vi "LEDpoi_main.vi"() -> ()   [LabVIEW 2014]
uses:
  typeDefs/location.ctl
  typeDefs/playParams.ctl
  typeDefs/editControl.ctl
  typeDefs/variantFlat.ctl
  typeDefs/editViewPlay.ctl
  typeDefs/loopDataType.ctl
  typeDefs/pictChooser.ctl
  typeDefs/labelInfo.ctl
  typeDefs/jumpTpInfo.ctl
  typeDefs/dimmerInfo.ctl
  typeDefs/cmdQaction.ctl
  typeDefs/pixxelAction.ctl
  <vilib>/Utility/sysdir.llb/System Directory Type.ctl
  typeDefs/parseAction.ctl
  typeDefs/saveDataType.ctl
  typeDefs/pixxelMultiAction.ctl
  <vilib>/picture/picture.llb/Draw True-Color Pixmap.vi
  <userlib>/_OpenG.lib/comparison/comparison.llb/U32 Changed__ogtk.vi
  <vilib>/Utility/file.llb/Read From Spreadsheet File (string).vi
  <userlib>/_OpenG.lib/array/array.llb/Empty 2D Array (String)__ogtk.vi
  <vilib>/Utility/file.llb/Write To Spreadsheet File (string).vi
  <vilib>/Utility/config.llb/NI_LVConfig.lvlib
panel:
  in  "debug":bool
  in  "loopData":T1
  in  "close":bool
  in  "mainTab":enum32{"editor", "Group", "setup", "unused1"}(tab)
  in  "delProg":bool
  in  "reloadProg":bool
  in  "openList":bool
  in  "saveList":bool
  in  "POI-Sequence":i32(listbox)
  in  "deleteProg":bool
  in  "loadProg":bool
  in  "saveProgAs":bool
  in  "activePoi":T5(radio) caption="Poi"
  in  "editArray":T2[](array[typedef])
  in  "editTab":enum32{"play", "LoopStart", "LoopEnd", "Dimmer"}(tab)
  out "Pixel":dbl
  out "2D Picture":picture
  in  "editDefPlay":T6={"delay"=100, "fromFrame"=0, "active"=TRUE, "picIndex"=2, "toFrame"=1, "loops"=0}
  out "Frame":dbl
  in  "labelInfo":T7={"LoopID"=1, "active"=TRUE, "LoopCount"=1} {"LoopCount" min=1 max=254; "LoopID" min=1 max=254}
  in  "loopEndInfo":T8={"LoopID"=1, "active"=TRUE} caption="Jump to..." {"LoopID" min=1 max=254}
  in  "dimmer":T9={"Dimmer Level"=100, "active"=TRUE} caption="Jump to..." {"Dimmer Level" min=1 max=254}
  in  "chooser":T4[](array[typedef])
  in  "uploadAll":bool
  in  "uploadProgOnly":bool
  in  "startProg":bool
  in  "pauseProg":bool
  out "error out":errorcluster
  in  "saveProg":bool
  out "working":bool
  out "status":string
  in  "jumpTo":bool
  in  "jumpi":u16(ring) caption="SyncPoint" items=["testprog1.poi"]
  out "Error":string
  in  "findMissing":bool
  in  "findAll":bool
  in  "startAll":bool
  in  "pauseAll":bool
  in  "jumpToAll":bool
  in  "jumpAllPt":u16(ring) caption="SyncPoint" items=["testprog1.poi"]
  out "activeTCP":bool[](array[boolean]) caption="active Pois"
  in  "erasePoi":bool
  in  "address":string="192.168.1.127" caption="Base Address"
  in  "connect":bool
  in  "exit":bool
  out "# elements":i32
  in  "AnzPois":i32=6
  out "code":u8[][](array[numeric])
  in  "reloadPNG":bool
  in  "fadeTime":u16
  out "60 x 30 Bitmap":u32[][](array[colorbox])
  in  "import PNG":bool
  in  "location":T10
  in  "playParams":T11={"startFrame"=0, "endFrame"=0, "loops"=1, "delayMSB"=60, "delayLSB"=10}
  in  "show":bool
  in  "black":bool
  in  "play":bool
  out "PNG":path
  # "shift - F5 for more ...."
  # "POIson V0.08 build 180328"
  # "Action List"
  # "Scenes"
  # "Program actions"
  # "Mouse over:"
  # "Loop Start"
  # "Loop End"
  # "Dimmer"
  # "[0-100%]"
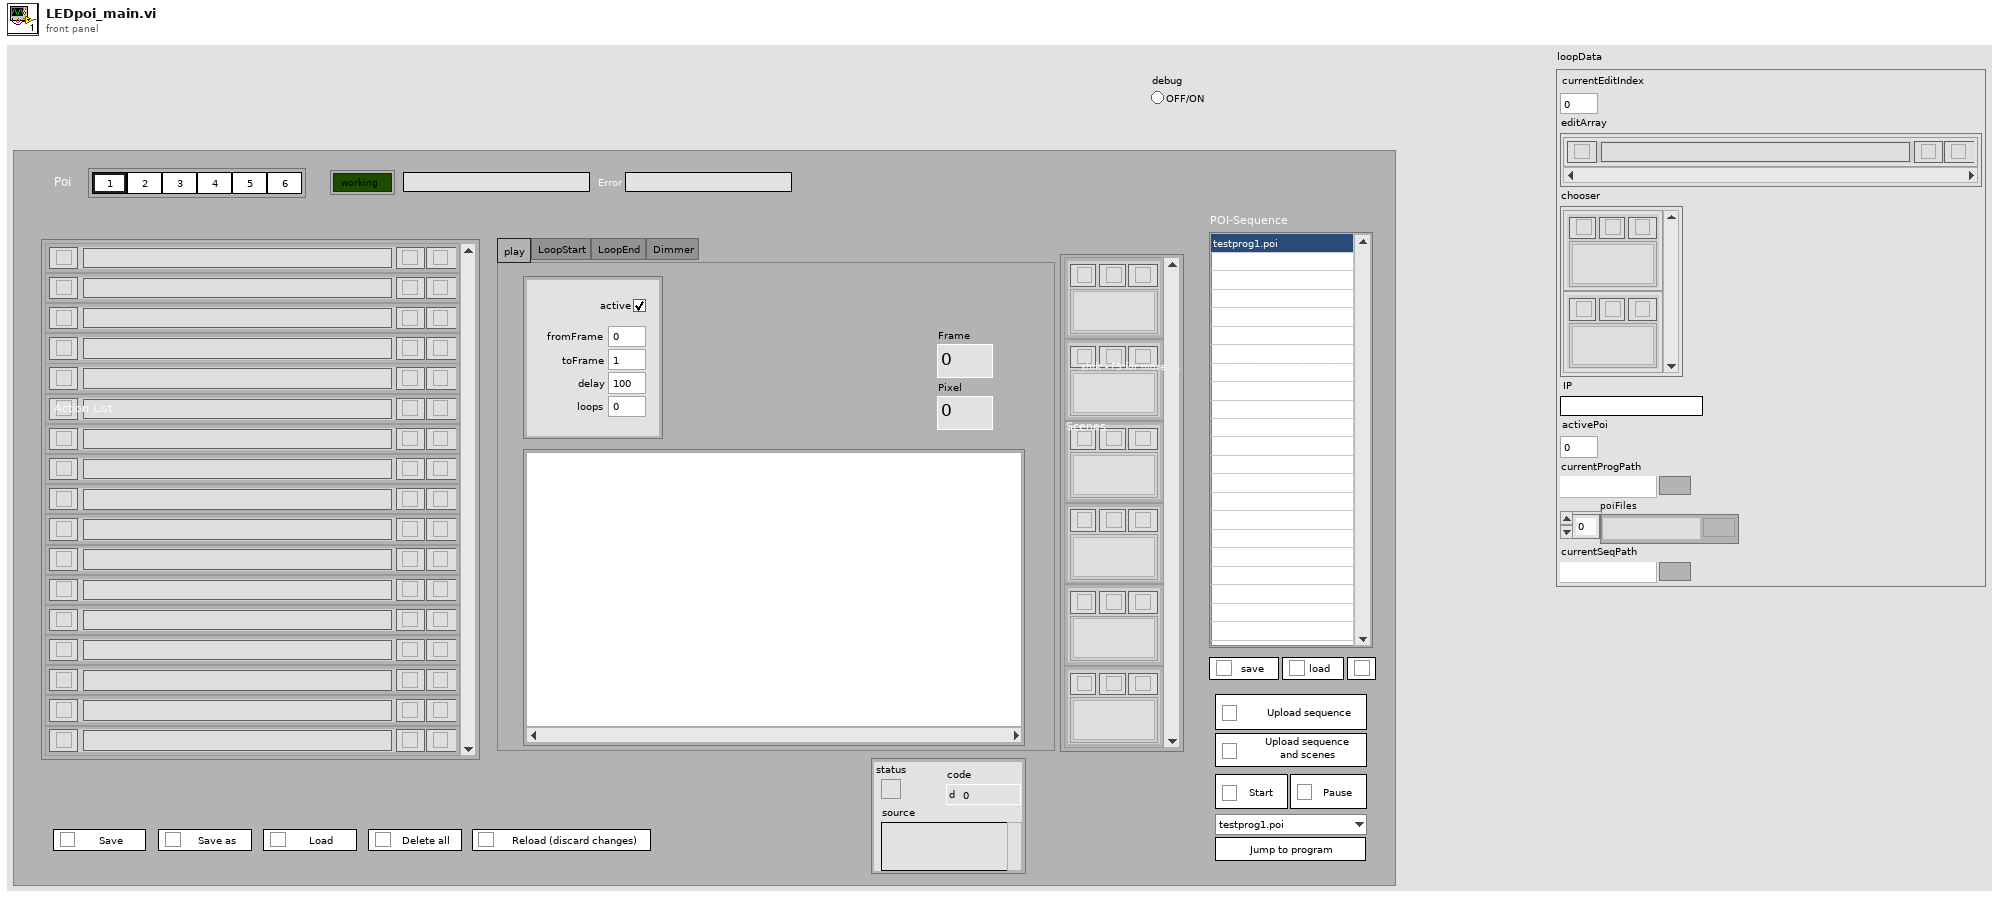
[diagram p1: front panel]
types:
  T1 = typedef "loopDataType.ctl" = cluster{"currentEditIndex":i32, "editArray":T2[], "chooser":T4[], "IP":string, "activePoi":i32, "currentProgPath":path, "poiFiles":path[], "currentSeqPath":path}
  T2 = typedef "editControl.ctl" = cluster{"edit":bool, "info":string, "variantFlat":T3, "codeCluster":cluster{"code":u8[][]}, "del":bool, "ins":bool}
  T3 = typedef "variantFlat.ctl" = cluster{"type string":i16[], "data string":string}
  T4 = typedef "pictChooser.ctl" = cluster{"2D Picture":picture, "load":bool, "Path":path, "Bitmap":u32[][], "del":bool, "paint":bool}
  T5 = enum32{"Radio Selection 1", "Radio Selection 2", "Radio Selection 3", "Radio Selection 4", "Radio Selection 5", "Radio Selection 6"}
  T6 = typedef "editViewPlay.ctl" = cluster{"delay":u16, "fromFrame":u8, "active":bool, "picIndex":i32, "toFrame":u8, "loops":u16}
  T7 = typedef "labelInfo.ctl" = cluster{"LoopID":u8, "active":bool, "LoopCount":u8}
  T8 = typedef "jumpTpInfo.ctl" = cluster{"LoopID":u8, "active":bool}
  T9 = typedef "dimmerInfo.ctl" = cluster{"Dimmer Level":u8, "active":bool}
  T10 = typedef "location.ctl" = cluster{"scene":u8, "frame":u8}
  T11 = typedef "playParams.ctl" = cluster{"startFrame":u8, "endFrame":u8, "loops":u8, "delayMSB":u8, "delayLSB":u8}
  T12 = typedef "cmdQaction.ctl" = enum16{"create", "enqueue", "getQueue"}
  T13 = typedef "pixxelMultiAction.ctl" = enum16{"init", "initAll", "initMissing", "watchdog", "black", "close", "startProg", "pauseProg", "stopProg", "jumpTo"}
  T14 = enum8{"Enabled", "Disabled", "Disabled and Grayed Out"}
  T15 = typedef "pixxelAction.ctl" = enum16{"init", "watchdog", "headScene", "setPixel", "tailScene", "headProg", "tailProg", "showSceneFrame", "black", "playFrames", "close", "uploadProg", "startProg", "pauseProg", "stopProg", "jumpTo", "setIP", "setGW", "initFlash", "saveScene", "saveProgram"}
  T16 = typedef "parseAction.ctl" = enum16{"play", "loopStart", "sync", "loopEnd", "dimm"}
  T17 = typedef "saveDataType.ctl" = cluster{"editArray":T2[], "bitmaps":cluster{"Bitmap":u32[][]}[], "paths":path[]}
  T18 = typedef "imagedata.ctl" = cluster{"image type":i32, "image depth":i32, "image":u8[], "mask":u8[], "colors":u32[], "Rectangle":cluster{"left":i16, "top":i16, "right":i16, "bottom":i16}}
  T19 = typedef "System Directory Type.ctl" = i32
  T20 = typedef "LVPoint32TypeDef.ctl" = cluster{"Horizontal":i32, "Vertical":i32}
  T21 = typedef "NI_LVConfig.lvlib/Config Data RefNum.ctl" = refnum<k1>
  T22 = enum32{"invalid app kind", "Development System", "Run Time System", "Student Edition", "Embedded LabVIEW", "Evaluation", "Custom"}
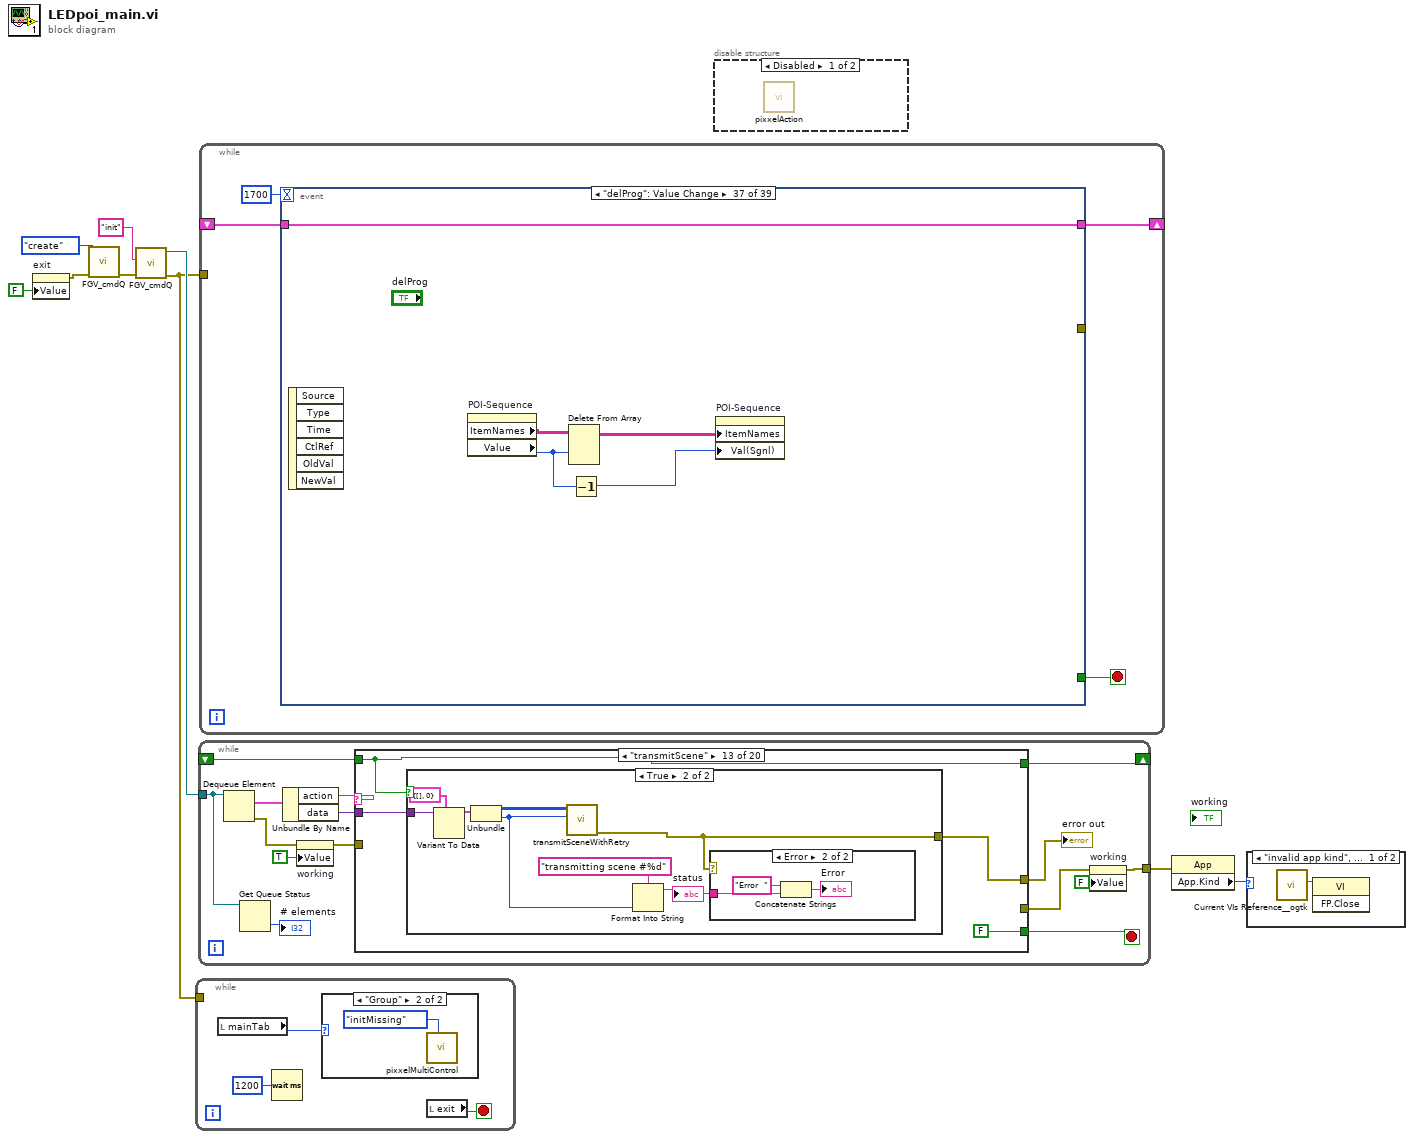
[diagram p0: block diagram]
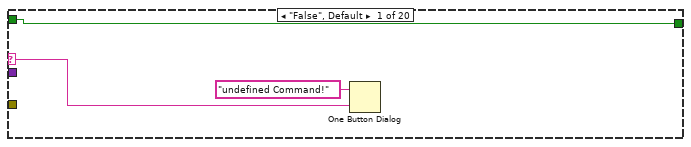
[diagram p4: hidden frame]
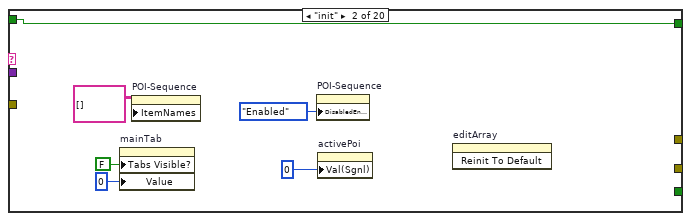
[diagram p5: hidden frame]
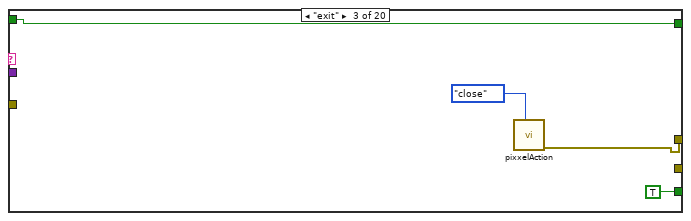
[diagram p6: hidden frame]
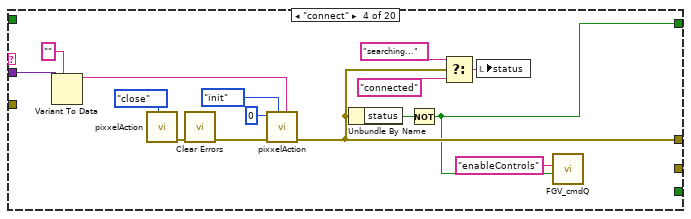
[diagram p7: hidden frame]
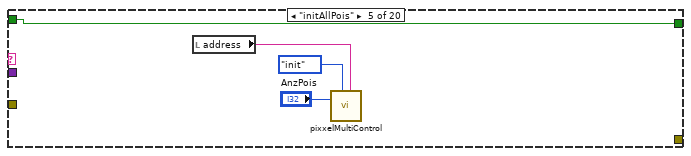
[diagram p8: hidden frame]
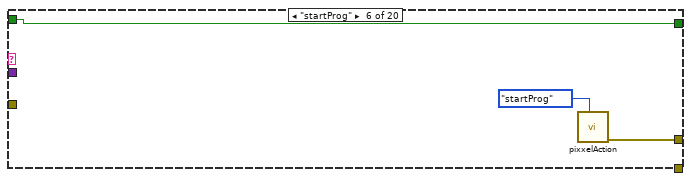
[diagram p9: hidden frame]
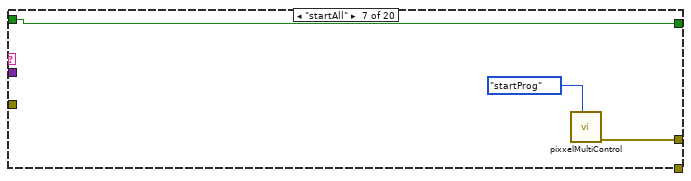
[diagram p10: hidden frame]
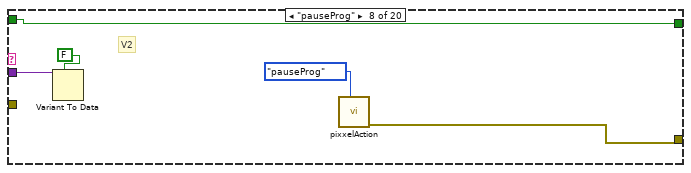
[diagram p11: hidden frame]
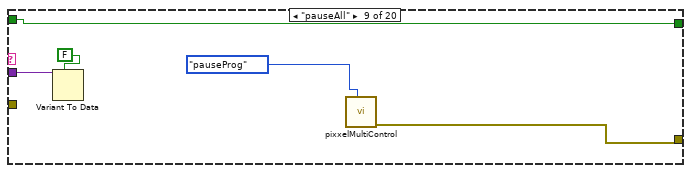
[diagram p12: hidden frame]
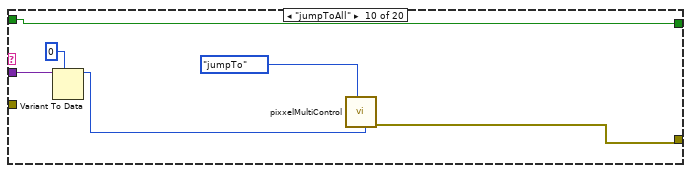
[diagram p13: hidden frame]
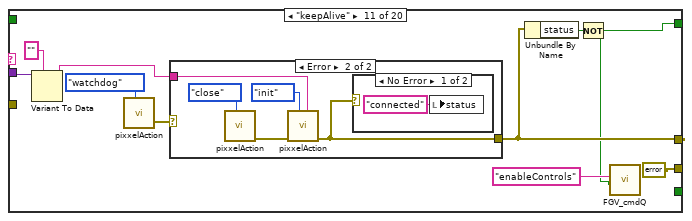
[diagram p14: hidden frame]
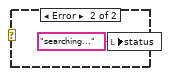
[diagram p16: hidden frame]
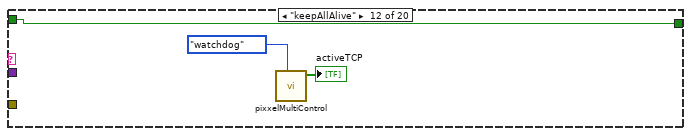
[diagram p17: hidden frame]
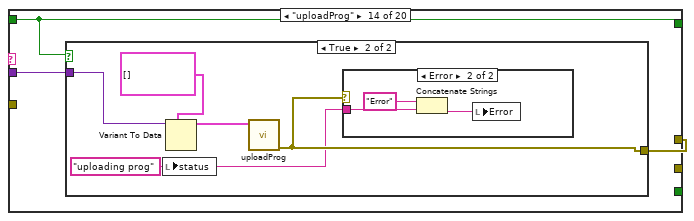
[diagram p20: hidden frame]
diagram:
  n1 = property on="exit" class="Bool (strict)"("Value"=FALSE ("exit")) -> (error out=w9:errorcluster)  [unwired: 2 in, 1 out]
  n2 = call "FGV_cmdQ.vi"("error in (no error)"=w9, "Qaction"=cmdQaction."create") -> ("error out"=w4:errorcluster)  [unwired: 8 in, 1 out]
  n3 = call "FGV_cmdQ.vi"("error in (no error)"=w4, "actionIn"="init") -> ("error out"=w2:errorcluster, "queue out"=w3:refnum<queue>)  [unwired: 8 in]
  n4 = while {
    tunnel: w2 -> [_]
    stop <- w12 stop-if-true
    n5 = local read "mainTab"() -> (w11:enum32{"editor", "Group", "setup", "unused1"})
    n6 = Wait (ms)(milliseconds to wait=u32 1200) -> ()  [unwired: 1 out]
    n7 = case shown="\"Group\"" w11 {
      frame "editor", Default {
      }
      frame "Group" {
        n8 = call "pixxelMultiControl.vi"("PIXXELaction"=pixxelMultiAction."initMissing") -> ()  [unwired: 9 in, 2 out]
      }
    }
    n9 = local read "exit"() -> (w12:bool)
  }
  n10 = while {
    tunnel: w3 -> [w17]
    shift-right: [w24] -> _
    shift-left: _ -> [w23]
    tunnel: [w19] -> w5
    stop <- w26 stop-if-true
    n11 = Dequeue Element(queue=w17) -> (element=w28:cluster{"action":string, "data":variant}, error out=w20:errorcluster)  [unwired: 2 in, 2 out]
    n12 = Get Queue Status(queue=w17) -> (# elements in queue=→"# elements":i32)  [unwired: 2 in, 7 out]
    n13 = Unbundle By Name(w28) -> ("action"=w27:string, "data"=w25:variant)
    n14 = property on="working" class="Bool (strict)"(error in=w20, "Value"=TRUE ("working")) -> (error out=w22:errorcluster)  [unwired: 1 in, 1 out]
    n15 = case shown="\"transmitScene\"" w27 {
      selector: w27 -> [w30 _ _ _ _ _ _ _ _ _ _ _ _ _ _ _ _ _ _ _]
      tunnel: [_ _ TRUE _ _ _ _ _ _ _ _ _ FALSE _ _ _ _ _ _ _] -> w26
      tunnel: w25 -> [_ _ _ w52 _ _ _ w69 w74 w79 w89 _ w105 w120 _ _ _ w141 w145 _]
      tunnel: [_ _ w38 w48 _ w62 w65 w68 w73 w81 w90 _ w104 w119 w129 _ _ _ _ w147] -> w15
      tunnel: [w29 w37 w40 w43 w60 w63 w66 w71 w76 w82 w83 w102 w103 w118 w131 w133 w135 w142 w146 w149] -> w24
      tunnel: w23 -> [w29 w37 w40 _ w60 w63 w66 w71 w76 w82 _ w102 w103 w118 w131 w133 w135 w142 w146 w149]
      tunnel: w22 -> [_ _ _ _ _ _ _ _ _ _ _ _ _ _ _ _ _ _ _ _]
      tunnel: [_ _ _ _ _ _ _ _ _ _ errorcluster {"status"=FALSE, "code"=0, "source"=""} ("error constant") _ _ _ _ _ _ _ _ _] -> w14
      frame "False", Default {
        n16 = One Button Dialog(message="undefined Command!", button name ("OK")=w30) -> ()  [unwired: 1 out]
      }
      frame "init" {
        n17 = property on="mainTab" class="TabCtl (strict)"("Tabs Visible?"=FALSE, "Value"=0) -> ()  [unwired: 2 in, 2 out]
        n18 = property on="POI-Sequence" class="MCListbox (strict)"("ItemNames"=string[][] []) -> ()  [unwired: 2 in, 2 out]
        n19 = property on="POI-Sequence" class="MCListbox (strict)"("DisabledEnum"=T14."Enabled" ("Disabled")) -> ()  [unwired: 2 in, 2 out]
        n20 = property on="activePoi" class="RadioBtnsControl (strict)"("Val(Sgnl)"=0) -> ()  [unwired: 2 in, 2 out]
        n21 = invoke on="editArray" class="Arr" method="Reinit To Default"() -> ()  [unwired: 3 in, 3 out]
      }
      frame "exit" {
        n22 = call "pixxelAction.vi"("PIXXELaction"=pixxelAction."close") -> ("error out"=w38:errorcluster)  [unwired: 10 in]
      }
      frame "connect" {
        n23 = Variant To Data(type="", Variant=w52) -> (data=w50:string)  [unwired: 1 in, 1 out]
        n24 = call "pixxelAction.vi"("PIXXELaction"=pixxelAction."close") -> ("error out"=w55:errorcluster)  [unwired: 10 in]
        n25 = call <vilib>:"Clear Errors.vi"("error in (no error)"=w55) -> ("error out"=w42:errorcluster)  [unwired: 5 in, 1 out]
        n26 = call "pixxelAction.vi"("address"=w50, "PIXXELaction"=pixxelAction."init", "error in (no error)"=w42, "Pixel-nummer"=u8 0 ("Pixel")) -> ("error out"=w48:errorcluster)  [unwired: 7 in]
        n27 = Unbundle By Name(w48) -> ("status"=w49:bool)
        n28 = Not(x=w49) -> (.not. x?=w43:bool)
        n29 = Select(t="searching..." ("status"), s=w48, f="connected" ("status")) -> (s? t:f=w45:string)
        n30 = local write "status"(w45) -> ()
        n31 = call "FGV_cmdQ.vi"("dataIn"=w43, "actionIn"="enableControls") -> ()  [unwired: 8 in, 2 out]
      }
      frame "initAllPois" {
        n32 = local read "address"() -> (w57:string)
        n33 = call "pixxelMultiControl.vi"("baseAddress"=w57, "PIXXELaction"=pixxelMultiAction."init", "AnzPois"="AnzPois") -> ()  [unwired: 7 in, 2 out]
      }
      frame "startProg" {
        n34 = call "pixxelAction.vi"("PIXXELaction"=pixxelAction."startProg") -> ("error out"=w62:errorcluster)  [unwired: 10 in]
      }
      frame "startAll" {
        n35 = call "pixxelMultiControl.vi"("PIXXELaction"=pixxelMultiAction."startProg") -> ("error out"=w65:errorcluster)  [unwired: 9 in, 1 out]
      }
      frame "pauseProg" {
        # "V2"
        n36 = Variant To Data(type=FALSE, Variant=w69) -> ()  [unwired: 1 in, 2 out]
        n37 = call "pixxelAction.vi"("PIXXELaction"=pixxelAction."pauseProg") -> ("error out"=w68:errorcluster)  [unwired: 10 in]
      }
      frame "pauseAll" {
        n38 = Variant To Data(type=FALSE, Variant=w74) -> ()  [unwired: 1 in, 2 out]
        n39 = call "pixxelMultiControl.vi"("PIXXELaction"=pixxelMultiAction."pauseProg") -> ("error out"=w73:errorcluster)  [unwired: 9 in, 1 out]
      }
      frame "jumpToAll" {
        n40 = Variant To Data(type=u16 0 ("jumpi 2"), Variant=w79) -> (data=w77:u16)  [unwired: 1 in, 1 out]
        n41 = call "pixxelMultiControl.vi"("u16"=w77, "PIXXELaction"=pixxelMultiAction."jumpTo") -> ("error out"=w81:errorcluster)  [unwired: 8 in, 1 out]
      }
      frame "keepAlive" {
        n42 = Variant To Data(type="", Variant=w89) -> (data=w87:string)  [unwired: 1 in, 1 out]
        n43 = call "pixxelAction.vi"("PIXXELaction"=pixxelAction."watchdog") -> ("error out"=w92:errorcluster)  [unwired: 10 in]
        n44 = case shown="Error" w92 {
          tunnel: [_ w95] -> w90
          tunnel: w87 -> [_ w96]
          frame No Error {
          }
          frame Error {
            n45 = call "pixxelAction.vi"("PIXXELaction"=pixxelAction."close") -> ("error out"=w94:errorcluster)  [unwired: 10 in]
            n46 = call "pixxelAction.vi"("address"=w96, "PIXXELaction"=pixxelAction."init", "error in (no error)"=w94) -> ("error out"=w95:errorcluster)  [unwired: 8 in]
            n47 = case shown="No Error" w95 {
              frame No Error {
                n48 = local write "status"("connected" ("status")) -> ()
              }
              frame Error {
                n49 = local write "status"("searching..." ("status")) -> ()
              }
            }
          }
        }
        n50 = Unbundle By Name(w90) -> ("status"=w84:bool)
        n51 = Not(x=w84) -> (.not. x?=w83:bool)
        n52 = call "FGV_cmdQ.vi"("dataIn"=w83, "actionIn"="enableControls") -> ()  [unwired: 8 in, 2 out]
      }
      frame "keepAllAlive" {
        n53 = call "pixxelMultiControl.vi"("PIXXELaction"=pixxelMultiAction."watchdog") -> ("activeTCP"=→"activeTCP":bool[])  [unwired: 9 in, 1 out]
      }
      frame "transmitScene" {
        n54 = case shown="True" w103 {
          tunnel: w105 -> [_ w113]
          tunnel: [_ w107] -> w104
          frame False {
          }
          frame True {
            n55 = Variant To Data(type=cluster{"24-bit pixmap":u32[][], i32} {"24-bit pixmap"=[], 0} ("output cluster"), Variant=w113) -> (data=w112:cluster{"24-bit pixmap":u32[][], i32})  [unwired: 1 in, 1 out]
            n56 = Unbundle(w112) -> ("24-bit pixmap"=w111:u32[][], w109:i32)
            n57 = call "transmitSceneWithRetry.vi"("scene #"=w109, "24-bit pixmap"=w111) -> ("error out"=w107:errorcluster)  [unwired: 9 in]
            n58 = Format Into String(format string="transmitting scene #%d", w109) -> (resulting string=w108:string)  [unwired: 2 in, 1 out]
            "status" <- w108
            n59 = case shown="Error" w107 {
              tunnel: w108 -> [_ w117]
              frame No Error {
              }
              frame Error {
                n60 = Concatenate Strings("Error  " ("string"), w117) -> (→"Error":string)
              }
            }
          }
        }
      }
      frame "uploadProg" {
        n61 = case shown="True" w118 {
          tunnel: w120 -> [_ w125]
          tunnel: [_ w122] -> w119
          frame False {
          }
          frame True {
            w121 = "uploading prog" ("status")
            n62 = local write "status"(w121) -> ()
            n63 = Variant To Data(type=T2[] [] ("editArray"), Variant=w125) -> (data=w123:T2[])  [unwired: 1 in, 1 out]
            n64 = call "uploadProg.vi"("editArray"=w123) -> ("error out"=w122:errorcluster)  [unwired: 10 in]
            n65 = case shown="Error" w122 {
              tunnel: w121 -> [_ w126]
              frame No Error {
              }
              frame Error {
                n66 = Concatenate Strings("Error" ("Error"), w126) -> (w127:string)
                n67 = local write "Error"(w127) -> ()
              }
            }
          }
        }
      }
      frame "erasePoi" {
        n68 = call "pixxelAction.vi"("PIXXELaction"=pixxelAction."initFlash") -> ("error out"=w129:errorcluster)  [unwired: 10 in]
      }
      frame "initAll" {
        n69 = call "pixxelMultiControl.vi"("PIXXELaction"=pixxelMultiAction."initAll") -> ()  [unwired: 9 in, 2 out]
      }
      frame "initMissing" {
        n70 = call "pixxelMultiControl.vi"("PIXXELaction"=pixxelMultiAction."initMissing") -> ()  [unwired: 9 in, 2 out]
      }
      frame "enableControls" {
        n71 = Variant To Data(type=FALSE, Variant=w141) -> (data=w139:bool)  [unwired: 1 in, 1 out]
        n72 = Select(t=T14."Enabled" ("Disabled"), s=w139, f=T14."Disabled and Grayed Out" ("Disabled")) -> (s? t:f=w136:T14)
        n73 = property on="uploadProgOnly" class="Bool"("DisabledEnum"=w136) -> ()  [unwired: 2 in, 2 out]
        n74 = property on="uploadAll" class="Bool"("DisabledEnum"=w136) -> ()  [unwired: 2 in, 2 out]
        n75 = property on="startProg" class="Bool"("DisabledEnum"=w136) -> ()  [unwired: 2 in, 2 out]
        n76 = property on="pauseProg" class="Bool (strict)"("DisabledEnum"=w136) -> ()  [unwired: 2 in, 2 out]
      }
      frame "showStatus" {
        n77 = Variant To Data(type="", Variant=w145) -> (data=w143:string)  [unwired: 1 in, 1 out]
        n78 = local write "status"(w143) -> ()
      }
      frame "closeTCP" {
        n79 = call "pixxelAction.vi"("PIXXELaction"=pixxelAction."close") -> ("error out"=w147:errorcluster)  [unwired: 10 in]
      }
    }
    "error out" <- w15
    n80 = property on="working" class="Bool (strict)"(error in=w14, "Value"=FALSE ("working")) -> (error out=w19:errorcluster)  [unwired: 1 in, 1 out]
  }
  n81 = while {
    tunnel: w2 -> [_]
    shift-right: [w151] -> _
    shift-left: _ -> [w150]
    stop <- w153 stop-if-true
    n82 = event shown="[36] \"delProg\": Value Change" {
      selector: _ -> [_ _ _ _ _ _ _ _ _ _ _ _ _ _ _ _ _ _ _ _ _ _ _ _ _ _ _ _ _ _ _ _ _ _ _ _ _ _ _]
      dyn-events: _ -> [_ _ _ _ _ _ _ _ _ _ _ _ _ _ _ _ _ _ _ _ _ _ _ _ _ _ _ _ _ _ _ _ _ _ _ _ _ _ _]
      timeout: 1700 -> [_ _ _ _ _ _ _ _ _ _ _ _ _ _ _ _ _ _ _ _ _ _ _ _ _ _ _ _ _ _ _ _ _ _ _ _ _ _ _]
      tunnel: [_ _ _ _ _ _ _ _ _ _ _ _ _ _ _ _ _ _ _ _ _ _ _ _ _ _ _ _ _ _ _ _ _ _ _ _ _ "exit" _] -> w153
      tunnel: [_ _ _ _ _ w185 w190 w196 w209 w216 _ _ _ _ _ _ _ _ _ _ _ _ _ w554 w590 _ _ _ _ _ _ _ _ _ _ _ _ _ _] -> _
      tunnel: [w157 w165 w172 w178 w182 w183 w187 w192 w207 w212 w220 w223 w227 w243 w317 w324 w431 w453 w455 w473 w495 w517 w539 w553 w589 w611 w617 w620 w622 w625 w628 w632 w633 w658 w681 w689 w700 w701 w708] -> w151
      tunnel: w150 -> [w162 w165 w172 w178 w182 w183 w187 w192 w207 w212 w220 w223 w227 w244 w317 w327 w431 w453 w455 w474 w496 w518 w540 w552 w586 w611 w617 w620 w622 w625 w628 w632 w633 w659 w681 w688 w700 w704 w708]
      event "connect", "activePoi", "address": Value Change {
        n83 = event-data() -> ()  [unwired: 1 in, 2 out]
        n84 = String To IP(1:"address") -> (0:w161:u32)
        n85 = Add(x="activePoi", y=w161) -> (x+y=w160:u32)
        n86 = IP To String(1:TRUE ("dot notation? (F)"), 2:w160) -> (0:w155:string)
        n87 = Bundle By Name(cluster=w162, "activePoi"="activePoi", "IP"=w155) -> (w157:T1)
        n88 = call "FGV_cmdQ.vi"("dataIn"=w155, "actionIn"="connect") -> ()  [unwired: 8 in, 2 out]
      }
      event "debug": Value Change {
        n89 = event-data() -> ()  [unwired: 1 in, 2 out]
        n90 = property on="mainTab" class="TabCtl (strict)"("Tabs Visible?"="debug", "Value"=0) -> ()  [unwired: 2 in, 2 out]
      }
      event Timeout {
        n91 = event-data() -> ()  [unwired: 1 in, 2 out]
        n92 = local read "mainTab"() -> (w166:enum32{"editor", "Group", "setup", "unused1"})
        n93 = Unbundle By Name(w172) -> ("IP"=w171:string)
        n94 = Equal To 0?(x=w166) -> (x = 0?=w170:bool)
        n95 = Select(t="keepAlive" ("actionIn"), s=w170, f="keepAllAlive" ("actionIn")) -> (s? t:f=w167:string)
        n96 = call "FGV_cmdQ.vi"("dataIn"=w171, "actionIn"=w167) -> ()  [unwired: 8 in, 2 out]
      }
      event "mainTab": Value Change {
        n97 = event-data() -> ()  [unwired: 1 in, 2 out]
        n98 = call "FGV_cmdQ.vi"("actionIn"="closeTCP") -> ("error out"=w176:errorcluster)  [unwired: 9 in, 1 out]
        n99 = call <userlib>:"wait_err.vi"("error in (no error)"=w176, "milliseconds to wait"=u32 100) -> ("error out"=w174:errorcluster)  [unwired: 9 in]
        n100 = case shown="\"Group\"" "mainTab" {
          tunnel: w174 -> [_ w179]
          frame "editor", Default {
          }
          frame "Group" {
            n101 = call "FGV_cmdQ.vi"("error in (no error)"=w179, "actionIn"="initAllPois") -> ()  [unwired: 8 in, 2 out]
          }
        }
      }
      event "close": Value Change {
        n102 = event-data() -> ()  [unwired: 1 in, 2 out]
        n103 = call "FGV_cmdQ.vi"("actionIn"="closeTCP") -> ()  [unwired: 9 in, 2 out]
      }
      event "show": Value Change {
        n104 = event-data() -> ()  [unwired: 1 in, 2 out]
        n105 = call "pixxelAction.vi"("PIXXELaction"=pixxelAction."showSceneFrame", "location"="location") -> ("error out"=w185:errorcluster)  [unwired: 9 in]
      }
      event "play": Value Change {
        n106 = event-data() -> ()  [unwired: 1 in, 2 out]
        n107 = local read "location"() -> (w189:T10)
        n108 = call "pixxelAction.vi"("playParams"="playParams", "PIXXELaction"=pixxelAction."playFrames", "location"=w189) -> ("error out"=w190:errorcluster)  [unwired: 8 in]
      }
      event "import PNG", "reloadPNG": Value Change {
        n109 = event-data() -> ()  [unwired: 1 in, 2 out]
        n110 = call <vilib>:"Set Busy.vi"() -> ("error out"=w198:errorcluster)  [unwired: 10 in, 1 out]
        n111 = local read "PNG"() -> (w194:path)
        n112 = case shown="True" "reloadPNG" {
          tunnel: [w203 w205] -> w200
          tunnel: w198 -> [w202 _]
          tunnel: [w201 w206] -> w195
          tunnel: w194 -> [_ w204]
          frame False {
            n113 = call <vilib>:"Read PNG File.vi"("error in (no error)"=w202) -> ("image data"=w203:T18, "path"=w201:path)  [unwired: 8 in, 1 out]
          }
          frame True {
            n114 = call <vilib>:"Read PNG File.vi"("path to PNG file"=w204) -> ("image data"=w205:T18, "path"=w206:path)  [unwired: 8 in, 1 out]
          }
        }
        "PNG" <- w195
        n115 = call <vilib>:"Unflatten Pixmap.vi"("image data"=w200) -> ("24-bit pixmap"=w199:u32[][])  [unwired: 4 in, 6 out]
        "60 x 30 Bitmap" <- w199
        n116 = call "transmitPicture.vi"("24-bit pixmap"=w199) -> ("error out"=w197:errorcluster)  [unwired: 10 in]
        n117 = call <vilib>:"Unset Busy.vi"("error in (no error)"=w197) -> ("error out"=w196:errorcluster)  [unwired: 10 in]
      }
      event "black": Value Change {
        n118 = event-data() -> ()  [unwired: 1 in, 2 out]
        n119 = call "pixxelAction.vi"("u16"="fadeTime", "PIXXELaction"=pixxelAction."black") -> ("error out"=w209:errorcluster)  [unwired: 9 in]
      }
      event "jumpTo": Value Change {
        n120 = event-data() -> ()  [unwired: 1 in, 2 out]
        n121 = Increment(x="jumpi") -> (x+1=w211:u16)
        n122 = Initialize Array(w211, 5 ("dimension size")) -> (w213:u16[])
        n123 = call "pixxelAction.vi"("inputArray"=w213, "PIXXELaction"=pixxelAction."jumpTo") -> ("error out"=w216:errorcluster)  [unwired: 9 in]
      }
      event "startProg": Value Change {
        n124 = event-data() -> ()  [unwired: 1 in, 2 out]
        n125 = local write "pauseProg"(FALSE ("pauseProg")) -> ()
        n126 = call "FGV_cmdQ.vi"("actionIn"="startProg") -> ()  [unwired: 9 in, 2 out]
      }
      event "pauseProg": Value Change {
        n127 = event-data() -> ()  [unwired: 1 in, 2 out]
        n128 = call "FGV_cmdQ.vi"("dataIn"="pauseProg", "actionIn"="pauseProg") -> ()  [unwired: 8 in, 2 out]
      }
      event "uploadAll", "uploadProgOnly": Value Change {
        n129 = event-data() -> ()  [unwired: 1 in, 2 out]
        n130 = property on="POI-Sequence" class="MCListbox (strict)"() -> ("ItemNames"=w226:string[][])  [unwired: 2 in, 2 out]
        n131 = call "fixPoiPaths.vi"("ItemNames"=w226, "loopData"=w227) -> ("ok"=w224:bool, "newPaths"=w225:path[])  [unwired: 8 in]
        n132 = local write "Error"("" ("Error")) -> ()
        n133 = case shown="True" w224 {
          tunnel: "uploadProgOnly" -> [_ w234]
          tunnel: w227 -> [_ w232]
          tunnel: w225 -> [_ w231]
          frame False {
            n134 = One Button Dialog(message="POI files missing.\nPlease move all *.poi-files\ninto the same folder als the *.seq") -> ()  [unwired: 1 in, 1 out]
          }
          frame True {
            n135 = Bundle By Name(cluster=w232, "poiFiles"=w231) -> (w235:T1)
            n136 = call "prepareUpload.vi"("progOnly"=w234, "loopData"=w235) -> ("code"=→"code":u8[][])  [unwired: 9 in]
          }
        }
      }
      event "editArray": Value Change {
        n137 = event-data() -> ()  [unwired: 1 in, 2 out]
        n138 = for {
          tunnel: "editArray" -> [w308] mode=indexing
          tunnel: [w314] -> w239
          tunnel: [w306] -> w245
          tunnel: [w313] -> w242
          tunnel: [w310] -> w241
          tunnel: [w309] -> w240 mode=indexing
          tunnel: [w305] -> w238
          tunnel: [w304] -> w236
          i -> [w314]
          stop <- w307 stop-if-true
          n139 = Unbundle By Name(w308) -> ("info"=w313:string, "variantFlat.type string"=w312:i16[], "variantFlat.data string"=w311:string)  [unwired: 1 out]
          n140 = Unbundle By Name(w308) -> ("edit"=w306:bool, "del"=w305:bool, "ins"=w304:bool)
          n141 = Compound Arithmetic op=OR(w306, w305, w304) -> (w307:bool)
          n142 = Flattened String To Variant(6:w311, 7:w312) -> (0:w309:errorcluster, 3:w310:variant)  [unwired: 1 in]
        }
        n143 = case shown="True" w245 {
          tunnel: w244 -> [w254 w275]
          tunnel: [w249 w281] -> w243
          tunnel: w239 -> [w247 w280]
          tunnel: w242 -> [_ w279]
          tunnel: w241 -> [_ w276]
          tunnel: w240 -> [_ _]
          tunnel: w238 -> [w253 _]
          tunnel: "editArray" -> [w252 _]
          tunnel: w236 -> [w250 _]
          frame False {
            n144 = case shown="False" w253 {
              tunnel: w247 -> [w256 w271]
              tunnel: w252 -> [w258 w273]
              tunnel: [w257 w272] -> w251
              tunnel: w250 -> [w259 _]
              tunnel: [w255 w270] -> w246
              frame False {
                n145 = case shown="False" w259 {
                  tunnel: w256 -> [w260 w262]
                  tunnel: w258 -> [w261 w264]
                  tunnel: [w261 w266] -> w257
                  tunnel: [w260 w262] -> w255
                  frame False {
                  }
                  frame True {
                    # "Insert"
                    n146 = Array Size(array=w264) -> (size(s)=w269:i32)
                    n147 = Decrement(x=w269) -> (x-1=w263:i32)
                    n148 = Greater Or Equal?(x=w262, y=w263) -> (x >= y?=w268:bool)
                    n149 = Insert Into Array(array=w264, index=w262, new element=T2 {"edit"=FALSE, "info"="", "variantFlat"={"type string"=[], "data string"=""}, "codeCluster"={"code"=[]}, "del"=FALSE, "ins"=FALSE} ("new element/subarray")) -> (w267:T2[])
                    n150 = Select(t=w264, s=w268, f=w267) -> (s? t:f=w266:T2[])
                  }
                }
              }
              frame True {
                # "delete"
                n151 = Delete From Array(array=w273, length=1, index=w271) -> (array with subset deleted=w272:T2[])  [unwired: 1 out]
                n152 = Decrement(x=w271) -> (x-1=w270:i32)
              }
            }
            n153 = call "resetEditArrayButtons.vi"("editpos"=w246, "editArray"=w251) -> ("editOut"=w248:T2[])  [unwired: 9 in]
            n154 = Bundle By Name(cluster=w254, "currentEditIndex"=w246, "editArray"=w248) -> (w249:T1)
            n155 = local write "editArray"(w248) -> ()
          }
          frame True {
            n156 = Match Pattern(string=w279, regular expression=":") -> (before substring=w277:string)  [unwired: 1 in, 3 out]
            n157 = case shown="\"dimm\"" w277 {
              tunnel: w276 -> [_ w289 w294 w298 w302]
              tunnel: w275 -> [_ w288 _ _ _]
              frame "False", Default {
              }
              frame "play" {
                n158 = Unbundle By Name(w288) -> ("chooser"=w286:T4[])
                n159 = Variant To Data(type=T6 {"delay"=0, "fromFrame"=0, "active"=FALSE, "picIndex"=0, "toFrame"=0, "loops"=0} ("editDef"), Variant=w289) -> (data=w287:T6)  [unwired: 1 in, 1 out]
                n160 = Unbundle By Name(w287) -> ("picIndex"=w285:i32)
                n161 = local write "editDefPlay"(w287) -> ()
                n162 = Index Array(array=w286, index=w285) -> (element=w284:T4)
                n163 = Unbundle By Name(w284) -> ("2D Picture"=w282:picture)
                n164 = local write "editTab"(0) -> ()
                n165 = property on="2D Picture" class="Pict"("Value"=w282, "ZoomFactor"=sgl 10.0 ("Zoom Factor")) -> ()  [unwired: 2 in, 2 out]
              }
              frame "loopStart" {
                n166 = Variant To Data(type=T7 {"LoopID"=1, "active"=FALSE, "LoopCount"=1} ("labelInfo"), Variant=w294) -> (data=w292:T7)  [unwired: 1 in, 1 out]
                n167 = local write "labelInfo"(w292) -> ()
                n168 = local write "editTab"(1) -> ()
              }
              frame "loopEnd" {
                n169 = Variant To Data(type=T8 {"LoopID"=1, "active"=TRUE} ("jumptoInfo"), Variant=w298) -> (data=w297:T8)  [unwired: 1 in, 1 out]
                n170 = local write "loopEndInfo"(w297) -> ()
                n171 = local write "editTab"(2) -> ()
              }
              frame "dimm" {
                n172 = Variant To Data(type=T9 {"Dimmer Level"=1, "active"=TRUE} ("dimmer"), Variant=w302) -> (data=w300:T9)  [unwired: 1 in, 1 out]
                n173 = local write "dimmer"(w300) -> ()
                n174 = local write "editTab"(3) -> ()
              }
            }
            n175 = Bundle By Name(cluster=w275, "currentEditIndex"=w280) -> (w281:T1)
          }
        }
      }
      event "editArray": Mouse Down {
        n176 = event-data() -> ()  [unwired: 1 in, 2 out]
        n177 = local read "editArray"() -> (w316:T2[])
        n178 = for {
          tunnel: w316 -> [w320] mode=indexing
          tunnel: [w318] -> w315 mode=indexing
          n179 = Bundle By Name(cluster=w320, "edit"=FALSE) -> (w318:T2)
        }
        n180 = local write "editArray"(w315) -> ()
      }
      event "chooser": Value Change {
        n181 = event-data() -> ()  [unwired: 1 in, 1 out]
        n182 = for {
          tunnel: "chooser" -> [w408] mode=indexing
          tunnel: [w409] -> w325
          tunnel: [w406] -> w329
          tunnel: [w408] -> w328
          tunnel: [w405] -> w323
          tunnel: [w404] -> w322
          i -> [w409]
          stop <- w407 stop-if-true
          n183 = Unbundle By Name(w408) -> ("load"=w406:bool, "del"=w405:bool, "paint"=w404:bool)
          n184 = Compound Arithmetic op=OR(w406, w405, w404) -> (w407:bool)
        }
        n185 = case shown="True" w329 {
          tunnel: w328 -> [_ w377]
          tunnel: "chooser" -> [_ w382]
          tunnel: w325 -> [w331 w381]
          tunnel: w327 -> [w333 w379]
          tunnel: [w332 w378] -> w324
          tunnel: w323 -> [w334 _]
          tunnel: w322 -> [w330 _]
          frame False {
            n186 = case shown="True" w334 {
              tunnel: w333 -> [w337 w367]
              tunnel: [w335 w368] -> w332
              tunnel: w331 -> [w336 w358]
              tunnel: w330 -> [w338 _]
              frame False {
                n187 = case shown="True" w338 {
                  tunnel: w337 -> [w339 w343]
                  tunnel: w336 -> [_ w345]
                  tunnel: [w339 w342] -> w335
                  frame False {
                  }
                  frame True {
                    w350 = T19 9 items=["User Home"=0, "User Desktop"=1, "User Documents"=2, "User Application Data"=3, "User Preferences"=4, "User Temporary"=5, "Public Documents"=6, "Public Application Data"=7, "Public Preferences"=8, "Public Cache"=13, "System Core Libraries"=9, "System Installed Libraries"=10, "Application Files"=11, "Boot Volume Root"=12] ("system directory type")
                    n188 = Unbundle By Name(w343) -> ("chooser"=w344:T4[])
                    n189 = Index Array(array=w344, index=w345) -> (element=w348:T4)
                    n190 = Unbundle By Name(w348) -> ("Path"=w355:path)
                    n191 = Bundle By Name(cluster=w348, "paint"=FALSE) -> (w346:T4)
                    n192 = Path To String(path=w355) -> (string=w353:string)
                    n193 = call <vilib>:"Get System Directory.vi"("system directory type"=w350) -> ("system directory"=w349:path)  [unwired: 10 in]
                    n194 = Replace Array Subset(array=w344, new element=w346, index=w345) -> (w341:T4[])
                    n195 = Concatenate Strings("mspaint.exe \"" ("command line"), w353, "\"" ("string")) -> (w351:string)
                    n196 = local write "chooser"(w341) -> ()
                    n197 = call <vilib>:"System Exec.vi"("wait until completion? (T)"=FALSE, "working directory"=w349, "command line"=w351) -> ("error out"=w340:errorcluster)  [unwired: 5 in, 3 out]
                    n198 = Bundle By Name(cluster=w343, "chooser"=w341) -> (w342:T1)
                    n199 = call <vilib>:"Clear Errors.vi"("error in (no error)"=w340) -> ()  [unwired: 5 in, 2 out]
                  }
                }
              }
              frame True {
                w363 = u32[][] [] ("Bitmap")
                # "Gelöschte Bilder nicht aus Array entfernen,\nda sonst der Bezug zu den Szenen nicht mehr stimmt"
                n200 = Unbundle By Name(w367) -> ("chooser"=w361:T4[])
                n201 = Array Size(array=w361) -> (size(s)=w360:i32)
                n202 = Index Array(array=w361, index=w358) -> (element=w366:T4)
                n203 = call-poly <vilib>:"Draw Unflattened Pixmap.vi"("data (RGB format)"=w363) -> ("new picture"=w362:picture)  [unwired: 8 in]
                n204 = Decrement(x=w360) -> (x-1=w359:i32)
                n205 = Bundle By Name(cluster=w366, "2D Picture"=w362, "del"=FALSE, "Bitmap"=w363) -> (w364:T4)
                n206 = Equal?(x=w358, y=w359) -> (x = y?=w357:bool)
                n207 = case shown="True" w357 {
                  tunnel: [w373 w375] -> w369
                  tunnel: w364 -> [w372 _]
                  tunnel: w361 -> [w371 w376]
                  tunnel: w358 -> [w370 w374]
                  frame False {
                    n208 = Replace Array Subset(array=w371, new element=w372, index=w370) -> (w373:T4[])
                  }
                  frame True {
                    n209 = Delete From Array(array=w376, index=w374) -> (array with subset deleted=w375:T4[])  [unwired: 1 in, 1 out]
                  }
                }
                n210 = Bundle By Name(cluster=w367, "chooser"=w369) -> (w368:T1)
                n211 = local write "chooser"(w369) -> ()
              }
            }
          }
          frame True {
            n212 = call "File Dialog"("prompt"="PNG wählen", "pattern (all files)"="*.png") -> ("selected path"=w383:path, "exists"=w386:bool, "cancelled"=w385:bool, "error out"=w380:errorcluster)  [unwired: 10 in]
            n213 = Compound Arithmetic op=AND(w386, invert w385) -> (w384:bool)
            n214 = case shown="True" w384 {
              tunnel: w383 -> [_ w399]
              tunnel: w377 -> [_ w402]
              tunnel: w382 -> [_ w398]
              tunnel: w381 -> [_ w393]
              tunnel: w380 -> [_ _]
              tunnel: w379 -> [w389 w396]
              tunnel: [w389 w394] -> w378
              frame False {
              }
              frame True {
                n215 = call <vilib>:"Read PNG File.vi"("path to PNG file"=w399) -> ("image data"=w403:T18)  [unwired: 8 in, 2 out]
                n216 = call <vilib>:"Unflatten Pixmap.vi"("image data"=w403) -> ("24-bit pixmap"=w392:u32[][])  [unwired: 4 in, 6 out]
                n217 = Array Subset(array=w392, length (row)=30 ("length")) -> (w391:u32[][])  [unwired: 3 in]
                n218 = call-poly <vilib>:"Draw Unflattened Pixmap.vi"("data (RGB format)"=w391) -> ("new picture"=w401:picture)  [unwired: 8 in]
                n219 = Bundle By Name(cluster=w402, "2D Picture"=w401, "Bitmap"=w391, "load"=FALSE, "Path"=w399) -> (w397:T4)
                n220 = Replace Array Subset(array=w398, new element=w397, index=w393) -> (w395:T4[])
                n221 = local write "chooser"(w395) -> ()
                n222 = Bundle By Name(cluster=w396, "chooser"=w395) -> (w394:T1)
              }
            }
          }
        }
        n223 = property on="POI-Sequence" class="MCListbox (strict)"("DisabledEnum"=T14."Disabled and Grayed Out" ("Disabled")) -> ()  [unwired: 2 in, 2 out]
      }
      event "chooser": Mouse Up {
        n224 = event-data() -> ("Coords.Vertical"=w430:i32)  [unwired: 1 in]
        n225 = property on="chooser" class="Arr"() -> ("Top"=w422:i32, "Index Values"=w421:u32[])  [unwired: 2 in, 2 out]
        n226 = Subtract(x=w430, y=w422) -> (x-y=w423:i32)
        n227 = property on="pictChooser" class="Clust"() -> ("Height"=w429:u32)  [unwired: 2 in, 2 out]
        n228 = Index Array(array=w421) -> (element=w418:u32)  [unwired: 1 in]
        n229 = Quotient & Remainder(x=w423, y=w429) -> (x-y*floor(x/y)=w411:u32, floor(x/y)=w412:u32)
        n230 = In Range and Coerce(upper limit=u32 80 ("y"), x=w411, lower limit=u32 38 ("y")) -> (In Range?=w413:bool)  [unwired: 1 out]
        n231 = local read "editTab"() -> (w426:enum32{"play", "LoopStart", "LoopEnd", "Dimmer"})
        n232 = Add(x=w412, y=w418) -> (x+y=w415:u32)
        n233 = local read "chooser"() -> (w428:T4[])
        n234 = call-poly <userlib>:"Data Changed__ogtk.vi"("U32"=w418) -> ("Changed"=w417:bool)
        n235 = To Long Integer(number=w426) -> (32bit integer=w425:i32)
        n236 = Not(x=w417) -> (.not. x?=w416:bool)
        n237 = Equal To 0?(x=w425) -> (x = 0?=w420:bool)
        n238 = Index Array(array=w428, index=w415) -> (element=w427:T4)
        n239 = Unbundle By Name(w427) -> ("2D Picture"=w424:picture)
        n240 = Compound Arithmetic op=AND(w413, w420, w416) -> (w419:bool)
        n241 = case shown="True" w419 {
          tunnel: w424 -> [w434 _]
          tunnel: w415 -> [w432 _]
          frame True {
            n242 = property on="2D Picture" class="Pict"("Value"=w434, "ZoomFactor"=sgl 10.0 ("Zoom Factor")) -> ()  [unwired: 2 in, 2 out]
            n243 = property on="picIndex" class="DigNum (strict)"("Val(Sgnl)"=w432) -> ()  [unwired: 2 in, 2 out]
          }
          frame False {
          }
        }
      }
      event "2D Picture": Mouse Move {
        n244 = event-data() -> ("CtlRef"=w436:refnum<vi>, "Coords"=w452:T20)  [unwired: 1 in, 3 out]
        n245 = Unbundle By Name(w452) -> ("Horizontal"=w451:i32, "Vertical"=w442:i32)
        n246 = property on="2D Picture" class="Pict"() -> ("Left"=w450:i32, "Top"=w441:i32)  [unwired: 2 in, 2 out]
        n247 = Subtract(x=w451, y=w450) -> (x-y=w449:i32)
        n248 = Subtract(x=w442, y=w441) -> (x-y=w443:i32)
        n249 = Divide(x=w449, y=10 ("scaler")) -> (x/y=w447:dbl)
        n250 = property class="Pict"(reference=w436) -> ("Left"=w435:i16)  [unwired: 1 in, 2 out]
        n251 = Divide(x=w443, y=10 ("scaler")) -> (x/y=w445:dbl)
        n252 = Round Toward -Infinity(1:w447) -> (0:w446:dbl)
        n253 = Round Toward -Infinity(1:w445) -> (0:w440:dbl)
        n254 = Add(x=w446, y=w435) -> (x+y=→"Frame":dbl)
        n255 = Subtract(x=30.0, y=w440) -> (x-y=→"Pixel":dbl)
      }
      event "editTab": Value Change {
        n256 = event-data() -> ("NewVal"=w454:enum32{"play", "LoopStart", "LoopEnd", "Dimmer"})  [unwired: 1 in]
        n257 = case shown="\"LoopEnd\"" w454 {
          frame "play" {
            n258 = local read "editDefPlay"() -> (w456:T6)
            n259 = property on="editDefPlay" class="Clust (strict)"("Val(Sgnl)"=w456) -> ()  [unwired: 2 in, 2 out]
          }
          frame "LoopStart" {
            n260 = local read "labelInfo"() -> (w457:T7)
            n261 = property on="labelInfo" class="Clust (strict)"("Val(Sgnl)"=w457) -> ()  [unwired: 2 in, 2 out]
          }
          frame "LoopEnd" {
            n262 = local read "loopEndInfo"() -> (w458:T8)
            n263 = property on="jumptoInfo" class="Clust (strict)"("Val(Sgnl)"=w458) -> ()  [unwired: 2 in, 2 out]
          }
          frame "Dimmer" {
            n264 = local read "dimmer"() -> (w459:T9)
            n265 = property on="dimmer" class="Clust (strict)"("Val(Sgnl)"=w459) -> ()  [unwired: 2 in, 2 out]
          }
          frame Default {
          }
        }
      }
      event Value Change {
        n266 = event-data() -> ()  [unwired: 1 in, 2 out]
        n267 = Unbundle By Name(w474) -> ("editArray"=w472:T2[], "currentEditIndex"=w464:i32)
        n268 = call "parsePlayInfo.vi"("action"=parseAction."play", "variantInfo"="editDefPlay") -> ("editArray"=w461:T2)  [unwired: 9 in]
        n269 = Array Size(array=w472) -> (size(s)=w471:i32)
        n270 = Greater?(x=w471, y=w464) -> (0:w470:bool)
        n271 = case shown="False" w470 {
          tunnel: w461 -> [w476 w481]
          tunnel: [w475 w480] -> w469
          tunnel: w472 -> [w477 w479]
          tunnel: w464 -> [_ w478]
          frame False {
            n272 = Build Array (concatenate)(w477, w476) -> (w475:T2[])
          }
          frame True {
            n273 = Replace Array Subset(array=w479, new element=w481, index=w478) -> (w480:T2[])
          }
        }
        n274 = Index Array(array=w469, index=w464) -> (element=w468:T2)
        n275 = Bundle By Name(cluster=w468, "edit"=TRUE) -> (w465:T2)
        n276 = Replace Array Subset(array=w469, new element=w465, index=w464) -> (w466:T2[])
        n277 = Bundle By Name(cluster=w474, "editArray"=w469) -> (w473:T1)
        n278 = local write "editArray"(w466) -> ()
        n279 = property on="POI-Sequence" class="MCListbox (strict)"("DisabledEnum"=T14."Disabled and Grayed Out" ("Disabled")) -> ()  [unwired: 2 in, 2 out]
      }
      event Value Change {
        n280 = event-data() -> ()  [unwired: 1 in, 2 out]
        n281 = Unbundle By Name(w496) -> ("editArray"=w494:T2[], "currentEditIndex"=w486:i32)
        n282 = call "parsePlayInfo.vi"("action"=parseAction."loopStart", "variantInfo"="labelInfo") -> ("editArray"=w483:T2)  [unwired: 9 in]
        n283 = Array Size(array=w494) -> (size(s)=w493:i32)
        n284 = Greater?(x=w493, y=w486) -> (0:w492:bool)
        n285 = case shown="False" w492 {
          tunnel: w483 -> [w498 w503]
          tunnel: [w497 w502] -> w491
          tunnel: w494 -> [w499 w501]
          tunnel: w486 -> [_ w500]
          frame False {
            n286 = Build Array (concatenate)(w499, w498) -> (w497:T2[])
          }
          frame True {
            n287 = Replace Array Subset(array=w501, new element=w503, index=w500) -> (w502:T2[])
          }
        }
        n288 = Index Array(array=w491, index=w486) -> (element=w490:T2)
        n289 = Bundle By Name(cluster=w490, "edit"=TRUE) -> (w487:T2)
        n290 = Replace Array Subset(array=w491, new element=w487, index=w486) -> (w488:T2[])
        n291 = Bundle By Name(cluster=w496, "editArray"=w491) -> (w495:T1)
        n292 = local write "editArray"(w488) -> ()
        n293 = property on="POI-Sequence" class="MCListbox (strict)"("DisabledEnum"=T14."Disabled and Grayed Out" ("Disabled")) -> ()  [unwired: 2 in, 2 out]
      }
      event Value Change {
        n294 = event-data() -> ()  [unwired: 1 in, 2 out]
        n295 = Unbundle By Name(w518) -> ("editArray"=w516:T2[], "currentEditIndex"=w508:i32)
        n296 = call "parsePlayInfo.vi"("action"=parseAction."loopEnd", "variantInfo"="loopEndInfo") -> ("editArray"=w505:T2)  [unwired: 9 in]
        n297 = Array Size(array=w516) -> (size(s)=w515:i32)
        n298 = Greater?(x=w515, y=w508) -> (0:w514:bool)
        n299 = case shown="False" w514 {
          tunnel: w505 -> [w520 w525]
          tunnel: [w519 w524] -> w513
          tunnel: w516 -> [w521 w523]
          tunnel: w508 -> [_ w522]
          frame False {
            n300 = Build Array (concatenate)(w521, w520) -> (w519:T2[])
          }
          frame True {
            n301 = Replace Array Subset(array=w523, new element=w525, index=w522) -> (w524:T2[])
          }
        }
        n302 = Index Array(array=w513, index=w508) -> (element=w512:T2)
        n303 = Bundle By Name(cluster=w512, "edit"=TRUE) -> (w509:T2)
        n304 = Replace Array Subset(array=w513, new element=w509, index=w508) -> (w510:T2[])
        n305 = Bundle By Name(cluster=w518, "editArray"=w513) -> (w517:T1)
        n306 = local write "editArray"(w510) -> ()
        n307 = property on="POI-Sequence" class="MCListbox (strict)"("DisabledEnum"=T14."Disabled and Grayed Out" ("Disabled")) -> ()  [unwired: 2 in, 2 out]
      }
      event Value Change {
        n308 = event-data() -> ()  [unwired: 1 in, 2 out]
        n309 = Unbundle By Name(w540) -> ("editArray"=w538:T2[], "currentEditIndex"=w530:i32)
        n310 = call "parsePlayInfo.vi"("action"=parseAction."dimm", "variantInfo"="dimmer") -> ("editArray"=w527:T2)  [unwired: 9 in]
        n311 = Array Size(array=w538) -> (size(s)=w537:i32)
        n312 = Greater?(x=w537, y=w530) -> (0:w536:bool)
        n313 = case shown="False" w536 {
          tunnel: w527 -> [w542 w547]
          tunnel: [w541 w546] -> w535
          tunnel: w538 -> [w543 w545]
          tunnel: w530 -> [_ w544]
          frame False {
            n314 = Build Array (concatenate)(w543, w542) -> (w541:T2[])
          }
          frame True {
            n315 = Replace Array Subset(array=w545, new element=w547, index=w544) -> (w546:T2[])
          }
        }
        n316 = Index Array(array=w535, index=w530) -> (element=w534:T2)
        n317 = Bundle By Name(cluster=w534, "edit"=TRUE) -> (w531:T2)
        n318 = Replace Array Subset(array=w535, new element=w531, index=w530) -> (w532:T2[])
        n319 = Bundle By Name(cluster=w540, "editArray"=w535) -> (w539:T1)
        n320 = local write "editArray"(w532) -> ()
        n321 = property on="POI-Sequence" class="MCListbox (strict)"("DisabledEnum"=T14."Disabled and Grayed Out" ("Disabled")) -> ()  [unwired: 2 in, 2 out]
      }
      event "saveProgAs", "saveProg": Value Change {
        n322 = Unbundle By Name(w552) -> ("currentProgPath"=w551:path)
        n323 = event-data() -> ()  [unwired: 1 in, 2 out]
        n324 = call <vilib>:"Check if File or Folder Exists.vi"("path"=w551) -> ("file or folder exists?"=w550:bool)  [unwired: 8 in, 2 out]
        n325 = Compound Arithmetic op=OR(invert w550, "saveProgAs") -> (w548:bool)
        n326 = case shown="False" w548 {
          tunnel: [w558 w561] -> w556
          tunnel: [FALSE ("cancelled") w560] -> w555
          tunnel: w551 -> [w558 w559]
          frame False {
          }
          frame True {
            n327 = call "File Dialog2"("start path"=w559, "prompt"="Save program as...", "pattern (all files)"="*.poi", "pattern label"="Poi Program") -> ("selected path"=w561:path, "cancelled"=w560:bool)  [unwired: 8 in, 2 out]
          }
        }
        n328 = case shown="False" w555 {
          tunnel: w552 -> [w568 w584]
          tunnel: w556 -> [w567 _]
          tunnel: [w575 _] -> w554
          tunnel: [w566 w584] -> w553
          frame False {
            n329 = Unbundle By Name(w568) -> ("editArray"=w573:T2[], "chooser"=w571:T4[])
            n330 = Bundle By Name(cluster=w568, "currentProgPath"=w567) -> (w566:T1)
            n331 = call <vilib>:"Open Config Data.vi"("create file if necessary (T)"=TRUE, "configuration file path"=w567) -> ("refnum"=w578:T21)  [unwired: 7 in, 2 out]
            n332 = for {
              tunnel: w571 -> [w583] mode=indexing
              tunnel: [w581] -> w570 mode=indexing
              tunnel: [w580] -> w569 mode=indexing
              n333 = Unbundle By Name(w583) -> ("Bitmap"=w582:u32[][], "Path"=w580:path)
              n334 = Bundle("Bitmap"=w582) -> (w581:cluster{"Bitmap":u32[][]})  [unwired: 1 in]
            }
            n335 = Bundle By Name(cluster=T17 {"editArray"=[], "bitmaps"=[], "paths"=[]} ("saveData"), "editArray"=w573, "bitmaps"=w570, "paths"=w569) -> (w572:T17)
            n336 = property on="POI-Sequence" class="MCListbox (strict)"("DisabledEnum"=T14."Enabled" ("Disabled")) -> ()  [unwired: 2 in, 2 out]
            n337 = call <userlib>:"Write INI Cluster__ogtk.vi"("INI Fomatted Cluster"=w572, "refnum"=w578) -> ("error out"=w577:errorcluster, "dup refnum"=w576:T21)  [unwired: 8 in]
            n338 = call <vilib>:"Close Config Data.vi"("error in (no error)"=w577, "refnum"=w576) -> ("error out"=w575:errorcluster)  [unwired: 8 in, 1 out]
          }
          frame True {
          }
        }
      }
      event "loadProg", "reloadProg": Value Change {
        n339 = event-data() -> ()  [unwired: 1 in, 2 out]
        n340 = case shown="False" "loadProg" {
          tunnel: [w593 w597] -> w592
          tunnel: [_ w596] -> w591
          tunnel: [_ w595] -> w588
          tunnel: w586 -> [w594 _]
          frame False {
            n341 = Unbundle By Name(w594) -> ("currentProgPath"=w593:path)
          }
          frame True {
            n342 = call "File Dialog3"("prompt"="Load program from...", "pattern (all files)"="*.poi", "pattern label"="Poi Program") -> ("selected path"=w597:path, "cancelled"=w596:bool, "error out"=w595:errorcluster)  [unwired: 9 in, 1 out]
          }
        }
        n343 = local write "loadProg"(FALSE ("loadProg")) -> ()
        n344 = case shown="False" w591 {
          tunnel: w586 -> [w605 w608]
          tunnel: w592 -> [w607 _]
          tunnel: [w606 _] -> w590
          tunnel: [w604 w608] -> w589
          tunnel: w588 -> [_ _]
          frame False {
            n345 = call "loadProg.vi"("selected path"=w607) -> ("error out"=w606:errorcluster, "scenes"=w601:T4[], "editArray"=w602:T2[])  [unwired: 8 in]
            n346 = local write "editArray"(w602) -> ()
            n347 = local write "chooser"(w601) -> ()
            n348 = property on="POI-Sequence" class="MCListbox (strict)"("DisabledEnum"=T14."Enabled" ("Disabled")) -> ()  [unwired: 2 in, 2 out]
            n349 = Bundle By Name(cluster=w605, "editArray"=w602, "chooser"=w601) -> (w604:T1)
          }
          frame True {
          }
        }
      }
      event "deleteProg": Value Change {
        n350 = event-data() -> ()  [unwired: 1 in, 2 out]
        n351 = Two Button Dialog(message="Delete current program?") -> (T button?=w609:bool)  [unwired: 2 in]
        n352 = case shown="True" w609 {
          frame False {
          }
          frame True {
            n353 = Initialize Array(T2 {"edit"=FALSE, "info"="", "variantFlat"={"type string"=[], "data string"=""}, "codeCluster"={"code"=[]}, "del"=FALSE, "ins"=FALSE} ("editCntrl"), 10 ("dimension size")) -> (w612:T2[])
            n354 = property on="editArray" class="Arr"("Val(Sgnl)"=w612) -> ()  [unwired: 2 in, 2 out]
          }
        }
      }
      event "erasePoi": Value Change {
        n355 = event-data() -> ()  [unwired: 1 in, 2 out]
        n356 = Two Button Dialog(message="Erase EVERYTHING in Poi Flash?") -> (T button?=w616:bool)  [unwired: 2 in]
        n357 = case shown="True" w616 {
          frame False {
          }
          frame True {
            n358 = call "FGV_cmdQ.vi"("actionIn"="erasePoi") -> ()  [unwired: 9 in, 2 out]
          }
        }
      }
      event "findAll": Value Change {
        n359 = event-data() -> ()  [unwired: 1 in, 2 out]
        n360 = call "FGV_cmdQ.vi"("actionIn"="initAll") -> ()  [unwired: 9 in, 2 out]
      }
      event "findMissing": Value Change {
        n361 = event-data() -> ()  [unwired: 1 in, 2 out]
        n362 = call "FGV_cmdQ.vi"("actionIn"="initMissing") -> ()  [unwired: 9 in, 2 out]
      }
      event "startAll": Value Change {
        n363 = event-data() -> ()  [unwired: 1 in, 2 out]
        n364 = local write "pauseAll"(FALSE ("pauseAll")) -> ()
        n365 = call "FGV_cmdQ.vi"("actionIn"="startAll") -> ()  [unwired: 9 in, 2 out]
      }
      event "pauseAll": Value Change {
        n366 = event-data() -> ()  [unwired: 1 in, 2 out]
        n367 = call "FGV_cmdQ.vi"("dataIn"="pauseAll", "actionIn"="pauseAll") -> ()  [unwired: 8 in, 2 out]
      }
      event "jumpToAll": Value Change {
        n368 = event-data() -> ()  [unwired: 1 in, 2 out]
        n369 = Increment(x="jumpAllPt") -> (x+1=w629:u16)
        n370 = call "FGV_cmdQ.vi"("dataIn"=w629, "actionIn"="jumpToAll") -> ()  [unwired: 8 in, 2 out]
      }
      event "POI-Sequence": Double Click {
        n371 = event-data() -> ("Row"=w635:i32)  [unwired: 1 in, 1 out]
        n372 = call "File Dialog4"("pattern (all files)"="*.poi", "pattern label"="Poi Sequence") -> ("selected path"=w634:path, "cancelled"=w636:bool)  [unwired: 10 in, 2 out]
        n373 = case shown="False" w636 {
          tunnel: w635 -> [w649 _]
          tunnel: w634 -> [w645 _]
          frame False {
            n374 = property on="POI-Sequence" class="MCListbox (strict)"() -> ("ItemNames"=w647:string[][])  [unwired: 2 in, 2 out]
            n375 = Strip Path(path=w645) -> (name=w643:string)  [unwired: 1 out]
            n376 = Path To String(path=w645) -> (string=w644:string)
            n377 = Array Size(array=w647) -> (size(s)=w650:i32[])
            n378 = Build Array(w643, w644) -> (w642:string[])
            n379 = Index Array(array=w650) -> (element=w646:i32)  [unwired: 1 in]
            n380 = Greater?(x=w646, y=w649) -> (0:w648:bool)
            n381 = case shown="True" w648 {
              tunnel: w647 -> [w652 w657]
              tunnel: w642 -> [w651 w654]
              tunnel: w649 -> [_ w655]
              tunnel: [w653 w656] -> w641
              frame False {
                n382 = Build Array (concatenate)(w652, w651) -> (w653:string[][])
              }
              frame True {
                n383 = Replace Array Subset(array=w657, new element=w654, index (row)=w655) -> (w656:string[][])  [unwired: 1 in]
              }
            }
            n384 = Index Array(array=w641, index (col)=0 ("disabled index (col)")) -> (element=w639:string[])  [unwired: 1 in]
            n385 = property on="POI-Sequence" class="MCListbox (strict)"("ItemNames"=w641) -> ()  [unwired: 2 in, 2 out]
            n386 = property on="jumpi" class="Ring (strict)"("Strings []"=w639) -> ()  [unwired: 2 in, 2 out]
            n387 = property on="jumpAllPt" class="Ring (strict)"("Strings []"=w639) -> ()  [unwired: 2 in, 2 out]
          }
          frame True {
          }
        }
      }
      event "openList": Value Change {
        n388 = event-data() -> ()  [unwired: 1 in, 6 out]
        n389 = call "File Dialog5"("pattern (all files)"="*.seq", "pattern label"="Sequence File") -> ("selected path"=w662:path, "cancelled"=w661:bool, "error out"=w660:errorcluster)  [unwired: 10 in, 1 out]
        n390 = case shown="False" w661 {
          tunnel: w662 -> [w667 _]
          tunnel: w660 -> [_ _]
          tunnel: w659 -> [w668 w675]
          tunnel: [w665 w675] -> w658
          frame False {
            n391 = Strip Path(path=w667) -> (stripped path=w666:path)  [unwired: 1 out]
            n392 = Bundle By Name(cluster=w668, "currentSeqPath"=w666) -> (w665:T1)
            n393 = call-poly <vilib>:"Read From Spreadsheet File.vi"("file path (dialog if empty)"=w667) -> ("all rows"=w670:string[][])  [unwired: 6 in, 4 out]
            n394 = call-poly <userlib>:"Empty Array__ogtk.vi"("Array"=w670) -> ("Empty Array?"=w669:bool)  [unwired: 8 in]
            n395 = case shown="False" w669 {
              tunnel: w670 -> [w674 _]
              frame False {
                n396 = property on="POI-Sequence" class="MCListbox (strict)"("ItemNames"=w674) -> ()  [unwired: 2 in, 2 out]
                n397 = Index Array(array=w674, index (col)=0 ("disabled index (col)")) -> (element=w672:string[])  [unwired: 1 in]
                n398 = property on="POI-Sequence" class="MCListbox (strict)"("Val(Sgnl)"=0 ("Value (Signaling)")) -> ()  [unwired: 2 in, 2 out]
                n399 = property on="jumpAllPt" class="Ring (strict)"("Strings []"=w672) -> ()  [unwired: 2 in, 2 out]
                n400 = property on="jumpi" class="Ring (strict)"("Strings []"=w672) -> ()  [unwired: 2 in, 2 out]
              }
              frame True {
              }
            }
          }
          frame True {
          }
        }
      }
      event "saveList": Value Change {
        n401 = event-data() -> ()  [unwired: 1 in, 6 out]
        n402 = call "File Dialog6"("pattern (all files)"="*.seq", "pattern label"="Sequence File") -> ("selected path"=w676:path, "cancelled"=w678:bool, "error out"=w677:errorcluster)  [unwired: 10 in, 1 out]
        n403 = case shown="False" w678 {
          tunnel: w677 -> [_ _]
          tunnel: w676 -> [w682 _]
          frame False {
            n404 = property on="POI-Sequence" class="MCListbox (strict)"() -> ("ItemNames"=w683:string[][])  [unwired: 2 in, 2 out]
            n405 = call-poly <vilib>:"Write To Spreadsheet File.vi"("2D data"=w683, "file path (dialog if empty)"=w682) -> ()  [unwired: 6 in, 1 out]
          }
          frame True {
          }
        }
      }
      event "POI-Sequence": Value Change {
        n406 = event-data() -> ()  [unwired: 1 in, 1 out]
        n407 = property on="POI-Sequence" class="MCListbox (strict)"() -> ("ItemNames"=w690:string[][])  [unwired: 2 in, 2 out]
        n408 = call "fixPoiPaths.vi"("ItemNames"=w690, "loopData"=w688) -> ("ok"=w687:bool, "newPaths"=w684:path[])  [unwired: 8 in]
        n409 = Index Array(array=w684, index="POI-Sequence") -> (element=w686:path)
        n410 = case shown="True" w687 {
          tunnel: w688 -> [w691 w693]
          tunnel: [w691 w695] -> w689
          tunnel: w686 -> [_ w692]
          frame False {
          }
          frame True {
            # "evil hack. VC with \"false\" disables file dialog\nin loadProg"
            n411 = property on="loadProg" class="Bool (strict)"("Val(Sgnl)"=FALSE ("Value (Signaling)")) -> ()  [unwired: 2 in, 2 out]
            n412 = Bundle By Name(cluster=w693, "currentProgPath"=w692) -> (w695:T1)
          }
        }
      }
      event "delProg": Value Change {
        n413 = event-data() -> ()  [unwired: 1 in, 6 out]
        n414 = property on="POI-Sequence" class="MCListbox (strict)"() -> ("ItemNames"=w699:string[][], "Value"=w697:i32)  [unwired: 2 in, 2 out]
        n415 = Delete From Array(array=w699, index (row)=w697) -> (array with subset deleted=w698:string[][])  [unwired: 2 in, 1 out]
        n416 = Decrement(x=w697) -> (x-1=w696:i32)
        n417 = property on="POI-Sequence" class="MCListbox (strict)"("ItemNames"=w698, "Val(Sgnl)"=w696) -> ()  [unwired: 2 in, 2 out]
      }
      event "exit": Value Change {
        # "type definition trick"
        n418 = event-data() -> ()  [unwired: 1 in, 2 out]
        n419 = Select(t=w704, s=TRUE, f="loopData") -> (s? t:f=w701:T1)
        n420 = call "FGV_cmdQ.vi"("actionIn"="exit") -> ()  [unwired: 9 in, 2 out]
      }
      event Panel Close? {
        w707 = TRUE ("Discard?")
        n421 = event-data() -> ()  [unwired: 1 in, 2 out]
        n422 = property on="exit" class="Bool (strict)"("Val(Sgnl)"=w707) -> ()  [unwired: 2 in, 2 out]
        n423 = event-data("Discard?"=w707) -> ()  [unwired: 1 in, 1 out]
      }
    }
  }
  n424 = disable-structure shown="Disabled" {
    frame Disabled {
      n425 = call "pixxelAction.vi"() -> ()  [unwired: 11 in, 1 out]
    }
    frame Enabled {
    }
  }
  n426 = property class="App"(error in=w5) -> ("App.Kind"=w6:T22)  [unwired: 1 in, 2 out]
  n427 = case shown="\"invalid app kind\", Default" w6 {
    frame "invalid app kind", Default {
      n428 = call <userlib>:"Current VIs Reference__ogtk.vi"() -> ("Current VI's reference"=w709:refnum<vi>)  [unwired: 5 in]
      n429 = invoke class="VI" method="FP.Close"(reference=w709) -> ()  [unwired: 2 in, 3 out]
    }
    frame "Development System" {
    }
  }
